vi "Write State.vi"(8 "error in (no error)":errorcluster, 10 "State":refnum<class "State Pattern.lvclass">, 11 "B Context State in":refnum<class "B Context State.lvclass">) -> (0 "error out":errorcluster, 3 "B Context State out":refnum<class "B Context State.lvclass">)   [LabVIEW 2021, in "Context.lvlib" / "B Context State.lvclass"]
uses:
  B Context State.lvclass
  State Pattern/State Pattern/State Pattern.lvclass
  Context/Context.lvclass
  B Context State.lvclass/B Context State.ctl
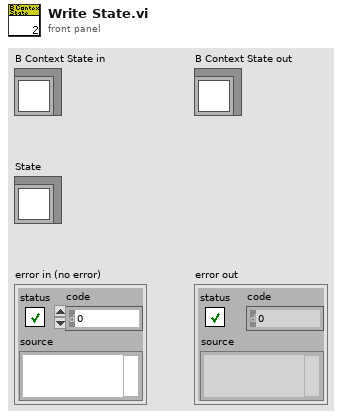
[diagram p1: front panel]
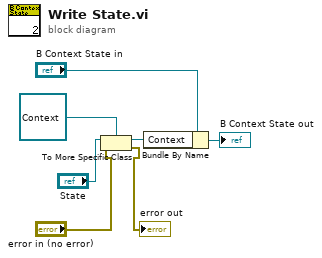
[diagram p0: block diagram]
diagram:
  n1 = To More Specific Class(target class=refnum<class "Context.lvclass"> refnum ("Context Actor.lvlib:Context Actor.lvclass"), reference="State", error in="error in (no error)") -> (specific class reference=w5:refnum<class "Context.lvclass">, error out=→"error out":errorcluster)
  n2 = Bundle By Name(cluster="B Context State in", "Context"=w5) -> (→"B Context State out":refnum<class "B Context State.lvclass">)
